vi "Teleop.vi"(10 "Match Info":T1={"Autonomous Elapsed Seconds"=0.0, "TeleOp Elapsed Seconds"=2239.335, "Disabled Elapsed Seconds"=2.9, "Visited Autonomous"=FALSE, "Visited TeleOp"=TRUE, "Visited Disabled"=TRUE, "Autonomous Settings"={"Autonomous Style"=enum."Independent", "VI Refnum"=refnum}}, 11 "Call Context":T2=enum."Stop") -> ()   [LabVIEW 2020]
doc: "This VI is called for each enabled TeleOp packet received from the DS. It is typically used to read from joysticks and other inputs and update I/O or setpoints for timed control loops. It should complete and return within 20 milliseconds or risk missing DS packets."
uses:
  <vilib>/Rock Robotics/WPI/DriverStation/WPI_DriverStationDerivedRobotMode.ctl
  <vilib>/Rock Robotics/WPI/DriverStation/WPI_DriverStationMatch Info.ctl
  <vilib>/Rock Robotics/WPI/Utilities/WPI_GetSetVariantRefNum.vi
  <vilib>/Rock Robotics/Network Tables/NT Write Boolean Array.vi
  <vilib>/Rock Robotics/Network Tables/NT Write Numeric Array.vi
panel:
  in  "Custom MaxTurnRateSlow (20)":dbl=20.0
  in  "Custom MaxTurnSlow (0.55)":dbl=0.55
  in  "Custom SlowRate (1)":dbl=1.0
  in  "Cheezy Drive Mode (2)":u16(ring)=1
  in  "Custom MaxSpeedSlow (0.6)":dbl=0.6
  in  "Quickturn":bool
  in  "CarLikeTurning":bool
  # "Cheezy Drive Settings"
  # "Enable to enable"
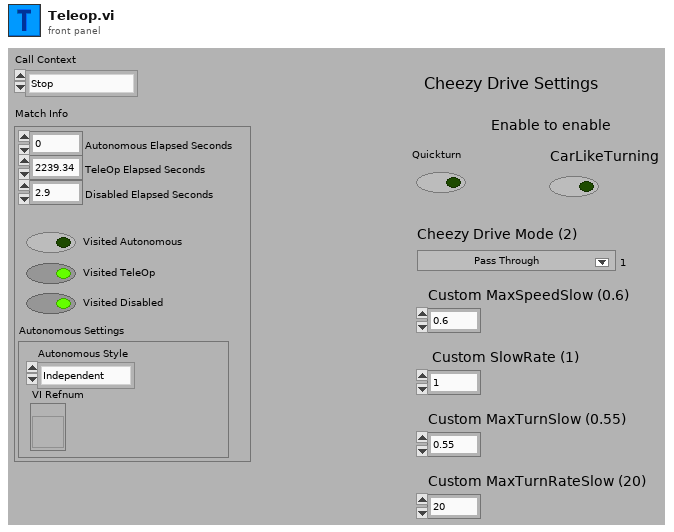
[diagram p1: front panel]
types:
  T1 = typedef "WPI_DriverStationMatch Info.ctl" = cluster{"Autonomous Elapsed Seconds":dbl, "TeleOp Elapsed Seconds":dbl, "Disabled Elapsed Seconds":dbl, "Visited Autonomous":bool, "Visited TeleOp":bool, "Visited Disabled":bool, "Autonomous Settings":cluster{"Autonomous Style":enum16{"Iterative", "Independent"}, "VI Refnum":refnum<vi>}}
  T2 = typedef "WPI_DriverStationDerivedRobotMode.ctl" = enum16{"Init", "Execute", "Stop"}
  T3 = typedef "WPI_JoystickDevRef.ctl" = cluster{"Device":T4}
  T4 = typedef "WPI_JoystickDeviceEnum.ctl" = enum16{"USB 0", "USB 1", "USB 2", "USB 3", "USB 4", "USB 5"}
  T5 = typedef "Command Status Info.ctl" = cluster{"Name":string, "Status":T6, "notifier out":T7}
  T6 = typedef "Completion Status.ctl" = enum16{"Successful", "Aborted", "Incomplete"}
  T7 = typedef "Completion Notifier.ctl" = refnum<notifier>
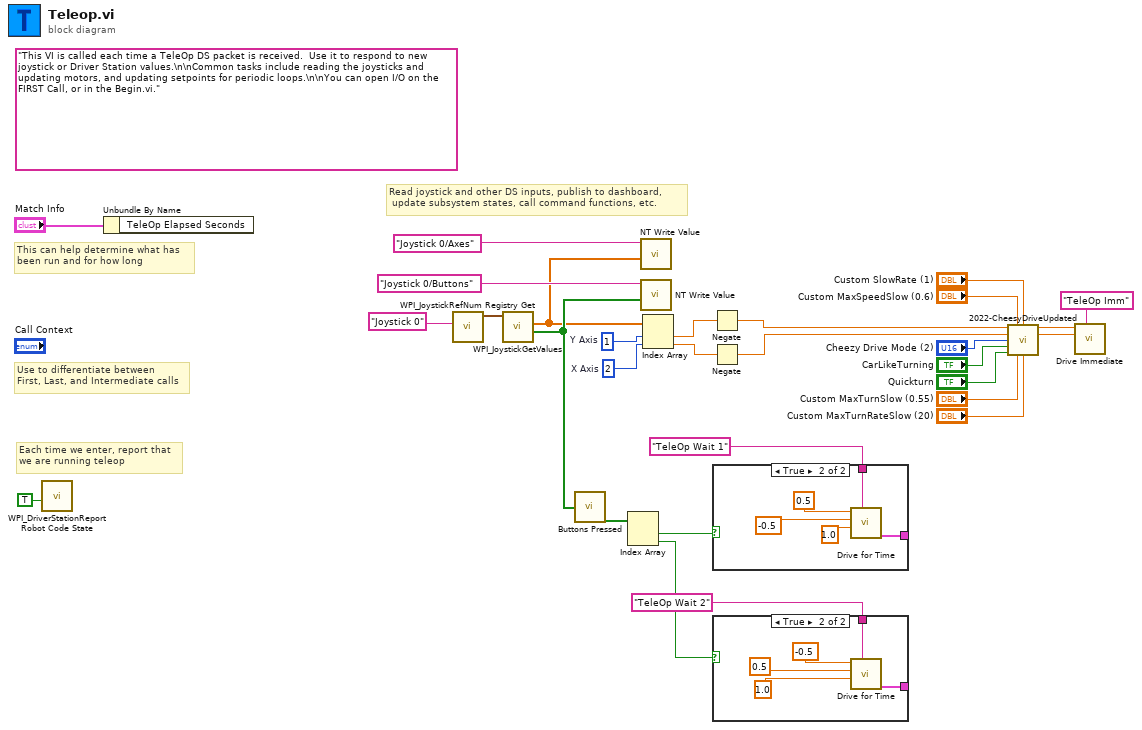
[diagram p0: block diagram]
diagram:
  w14 = 1  # Y Axis
  w13 = 2  # X Axis
  (unwired) "This VI is called each time a TeleOp DS packet is received.  Use it to respond to new joystick or Driver Station values.\n\nCommon tasks include reading the joysticks and updating motors, and updating setpoints for periodic loops.\n\nYou can open I/O on the FIRST Call, or in the Begin.vi."
  # "Read joystick and other DS inputs, publish to dashboard,\n update subsystem states, call command functions, etc."
  # "Each time we enter, report that\nwe are running teleop"
  # "Use to differentiate between\nFirst, Last, and Intermediate calls"
  # "This can help determine what has\nbeen run and for how long"
  n1 = call <vilib>:"WPI_DriverStationReport Robot Code State.vi"("TeleOp"=TRUE ("Autonomous")) -> ()  [unwired: 10 in, 1 out]
  n2 = Unbundle By Name("Match Info") -> ()  [unwired: 1 out]
  n3 = call <vilib>:"WPI_JoystickRefNum Registry Get.vi"("refnum name"="Joystick 0") -> ("JoystickDevRef"=w26:T3)  [unwired: 1 in, 9 out]
  n4 = call <vilib>:"WPI_JoystickGetValues.vi"("JoystickDevRef"=w26) -> ("Buttons"=w17:bool[], "Axes"=w16:dbl[])  [unwired: 6 in, 3 out]
  n5 = call "Buttons Pressed.vi"("Button Values"=w17) -> ("Button Presses"=w22:bool[])
  n6 = Index Array(array=w22) -> (element #1=w21:bool, element #2=w20:bool)  [unwired: 2 in]
  n7 = call-poly <vilib>:"NT Write Value.vi"("Numeric Array"=w16, "Name"="Joystick 0/Axes") -> ()  [unwired: 9 in, 1 out]
  n8 = call-poly <vilib>:"NT Write Value.vi"("Boolean Array"=w17, "Name"="Joystick 0/Buttons") -> ()  [unwired: 9 in, 1 out]
  n9 = Index Array(array=w16, index #1=w14, index #2=w13) -> (element #1=w12:dbl, element #2=w11:dbl)
  n10 = Negate(x=w12) -> (-x=w10:dbl)
  n11 = Negate(x=w11) -> (-x=w9:dbl)
  n12 = case shown="True" w21 {
    tunnel: [_ w33] -> _
    tunnel: "TeleOp Wait 1" ("Description") -> [_ w32]
    frame False {
    }
    frame True {
      n13 = call "Drive for Time.vi"("Description"=w32, "Seconds"=1.0, "Right Speed"=-0.5, "Left Speed"=0.5) -> ("Command Info Out"=w33:T5)  [unwired: 7 in]
    }
  }
  n14 = case shown="True" w20 {
    tunnel: [_ w37] -> _
    tunnel: "TeleOp Wait 2" ("Description") -> [_ w36]
    frame False {
    }
    frame True {
      n15 = call "Drive for Time.vi"("Description"=w36, "Seconds"=1.0, "Right Speed"=0.5, "Left Speed"=-0.5) -> ("Command Info Out"=w37:T5)  [unwired: 7 in]
    }
  }
  n16 = call "2022-CheesyDriveUpdated.vi"("Throttle"=w10, "Custom MaxSpeedSlow (0.6)"="Custom MaxSpeedSlow (0.6)", "Custom SlowRate (1)"="Custom SlowRate (1)", "Wheel"=w9, "Cheezy Drive Mode (2)"="Cheezy Drive Mode (2)", "CarLikeTurning"="CarLikeTurning", "Quickturn"="Quickturn", "Custom MaxTurnSlow (0.55)"="Custom MaxTurnSlow (0.55)", "Custom MaxTurnRateSlow (20)"="Custom MaxTurnRateSlow (20)") -> ("Left PWM"=w19:dbl, "Right PWM"=w8:dbl)  [unwired: 5 in]
  n17 = call "Drive Immediate.vi"("Description"="TeleOp Imm", "Right Setpoint"=w8, "Left Setpoint"=w19) -> ()  [unwired: 8 in, 1 out]
